vi "Lian_Lab02_I1.vi"() -> ()   [LabVIEW 2020]
uses:
  <vilib>/measure/NI_MABase.lvlib
panel:
  out "Iteration Count":i32
  in  "frequency":dbl=10.0 format="%0.2p"
  in  "amplitude":dbl=1.0 format="%0.2p"
  in  "phase":dbl format="%.2p"
  in  "sampling info":cluster{"Fs":dbl, "#s":dbl}={"Fs"=1000.0, "#s"=1000.0} {"Fs" format="%.2p"}
  in  "offset":dbl format="%0.2p"
  in  "Stop":bool
  out "Waveform Chart":waveform(dbl)(graph)
  out "Waveform Graph":waveform(dbl)(graph)
  # "Basic Waveform Chart While Loop"
  # "Note: Panel objects are locked . Unlock to access additional features."
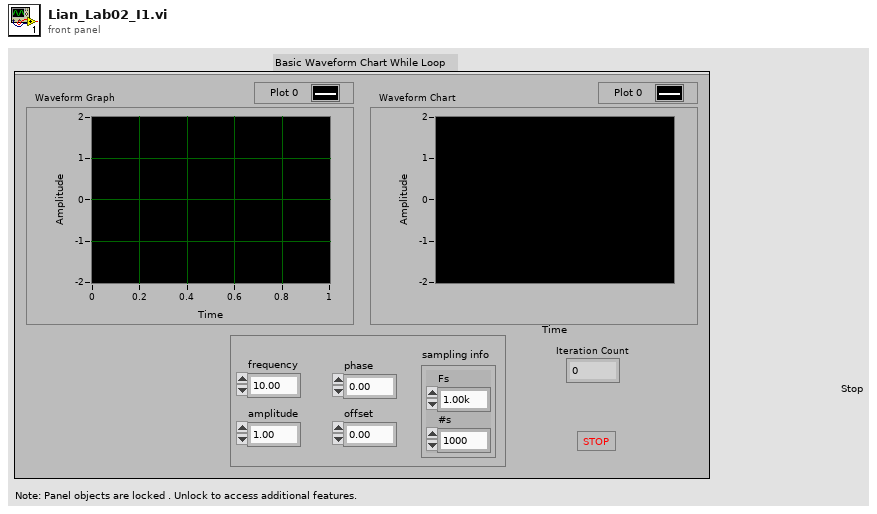
[diagram p1: front panel]
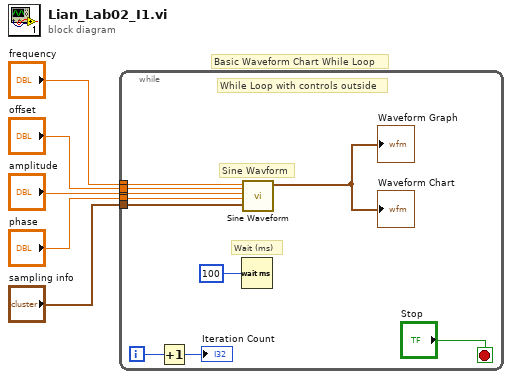
[diagram p0: block diagram]
diagram:
  # "Basic Waveform Chart While Loop"
  n1 = while {
    tunnel: "amplitude" -> [w15]
    tunnel: "frequency" -> [w14]
    tunnel: "offset" -> [w13]
    tunnel: "phase" -> [w12]
    tunnel: "sampling info" -> [w11]
    i -> [w7]
    stop <- "Stop" stop-if-true
    # "While Loop with controls outside"
    # "Wait (ms)"
    # "Sine Wavform"
    n2 = Increment(x=w7) -> (x+1=→"Iteration Count":i32)
    n3 = Wait (ms)(milliseconds to wait=u32 100) -> ()  [unwired: 1 out]
    n4 = call <vilib>:"Sine Waveform.vi"("offset"=w13, "sampling info"=w11, "phase"=w12, "amplitude"=w15, "frequency"=w14) -> ("signal out"=→"Waveform Graph" →"Waveform Chart":waveform(dbl))  [unwired: 5 in, 1 out]
  }
